vi "test_linear_interpolation.vi"() -> ()   [LabVIEW 2009]
doc: "Copyright (c) 2010 Stepan A. Baranov (stepan@baranov.su)\nAll rights reserved.\nweb-site: www.OCTLab.org"
uses:
  <vilib>/gmath/NI_Gmath.lvlib
  OCTLib_64.dll
panel:
  out "RSM_STAT final 2D array":dbl[](array[numeric])
  out "error out":errorcluster
  out "data Graph":dbl[][](graph)
  out "wavelengths Graph":dbl[][](graph)
  out "LabView final 2D array":dbl[](array[numeric])
  out "initial 2D array":dbl[](array[numeric])
  in  "stop":bool
  in  "index (row)":i32=1
  in  "Y":i32=9
  in  "X":i32=800
  in  "End wavelength":dbl=890.0
  in  "Start wavelength":dbl=800.0
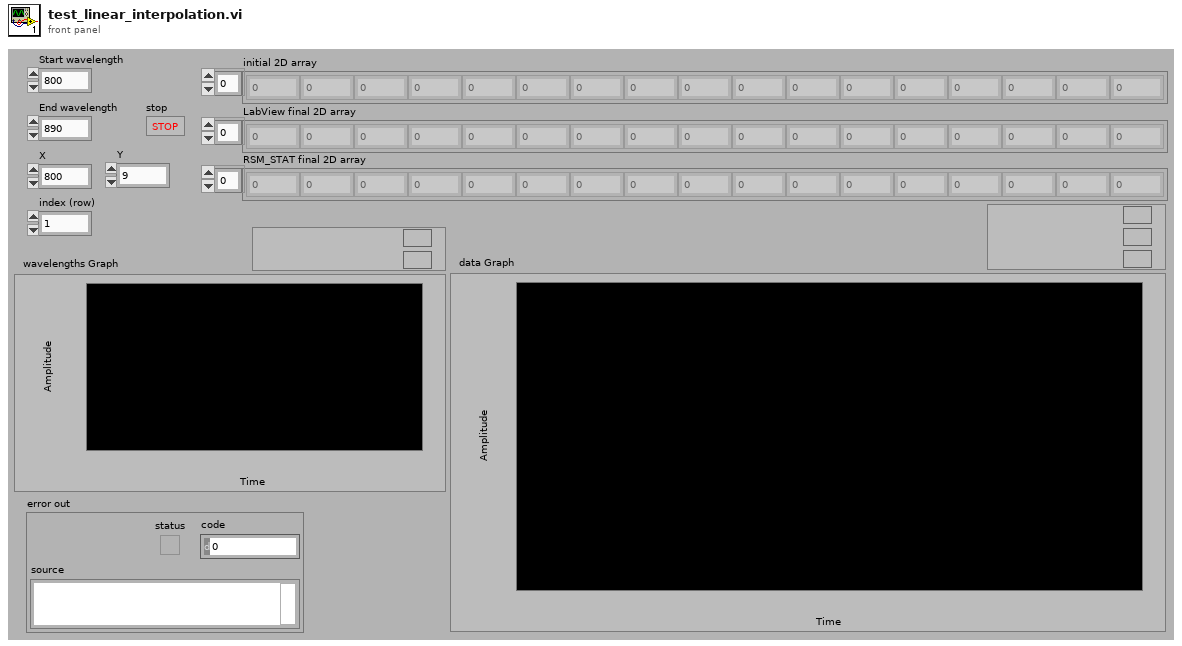
[diagram p1: front panel]
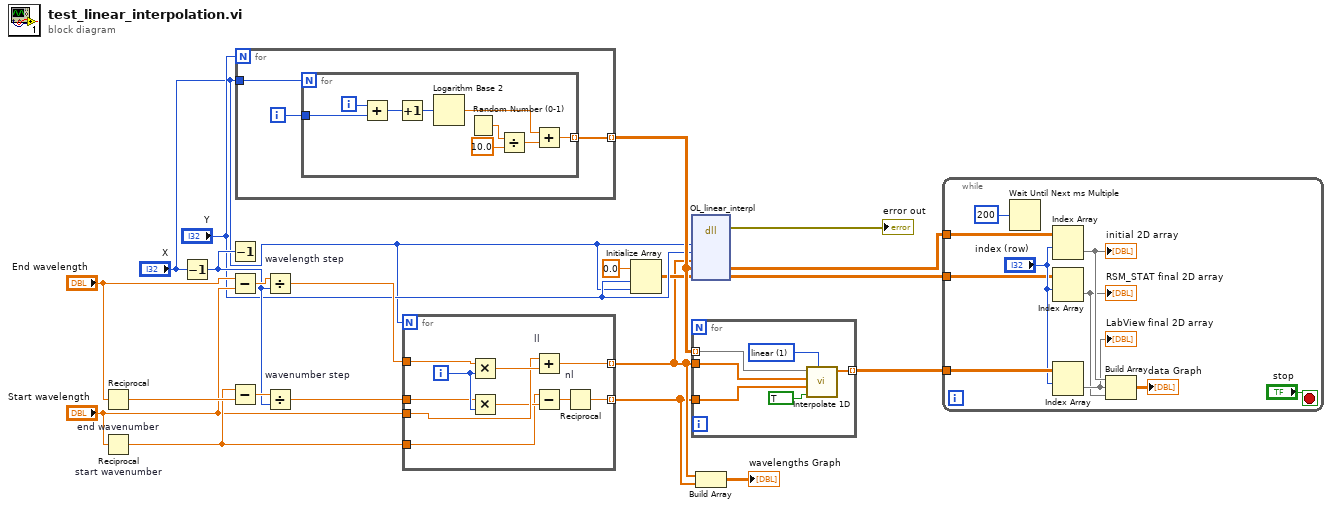
[diagram p0: block diagram]
diagram:
  n1 = Reciprocal "end wavenumber"(x="End wavelength") -> (1/x=w20:dbl)
  n2 = Reciprocal "start wavenumber"(x="Start wavelength") -> (1/x=w15:dbl)
  n3 = Decrement(x="X") -> (x-1=w18:i32)
  n4 = Decrement(x=w18) -> ()  [unwired: 1 out]
  n5 = Subtract(x="End wavelength", y="Start wavelength") -> (x-y=w21:dbl)
  n6 = Subtract(x=w15, y=w20) -> (x-y=w19:dbl)
  n7 = for {
    N: "Y" -> [_]
    tunnel: [w24] -> w11 mode=indexing
    tunnel: "X" -> [w23]
    i -> [w22]
    n8 = for {
      N: w23 -> [_]
      tunnel: [w25] -> w24 mode=indexing
      tunnel: w22 -> [w33]
      i -> [w32]
      n9 = Add(x=w32, y=w33) -> (x+y=w31:i32)
      n10 = Increment(x=w31) -> (x+1=w30:i32)
      n11 = Logarithm Base 2(1:w30) -> (0:w29:dbl)
      n12 = Random Number (0-1)() -> (number: 0 to 1=w28:dbl)
      n13 = Divide(x=w28, y=10.0) -> (x/y=w26:dbl)
      n14 = Add(x=w29, y=w26) -> (x+y=w25:dbl)
    }
  }
  n15 = Divide "wavelength step"(x=w21, y=w18) -> (x/y=w17:dbl)
  n16 = Divide "wavenumber step"(x=w19, y=w18) -> (x/y=w16:dbl)
  n17 = for {
    N: "X" -> [_]
    tunnel: w17 -> [w43]
    tunnel: "Start wavelength" -> [w41]
    tunnel: [w40] -> w3 mode=indexing
    tunnel: w16 -> [w38]
    tunnel: w15 -> [w35]
    tunnel: [w34] -> w2 mode=indexing
    i -> [w39]
    n18 = Multiply(x=w43, y=w39) -> (x*y=w42:dbl)
    n19 = Multiply(x=w38, y=w39) -> (x*y=w36:dbl)
    n20 = Add "ll"(x=w41, y=w42) -> (x+y=w40:dbl)
    n21 = Subtract(x=w35, y=w36) -> (x-y=w37:dbl)
    n22 = Reciprocal "nl"(x=w37) -> (1/x=w34:dbl)
  }
  n23 = Initialize Array(0.0 ("element"), "Y", "X") -> (w6:dbl[][])
  n24 = dll-call lib="OCTLib**.*" fn="OL_linear_interpl"("width"="X", "height"="Y", "spectrum"=w3, "in"=w11, "out"=w6) -> (error out=→"error out":errorcluster, "in"=w4:dbl[][], "out"=w10:dbl[][])  [unwired: 7 in, 1 out]
  n25 = for {
    tunnel: w11 -> [w49] mode=indexing
    tunnel: w3 -> [w48]
    tunnel: w2 -> [w47]
    tunnel: [w44] -> w1 mode=indexing
    w45 = 1 items=["nearest", "linear", "spline", "cubic Hermite", "Lagrange"] ("method")
    n26 = call <vilib>:"Interpolate 1D.vi"("method"=w45, "X is monotonic"=TRUE, "xi"=w47, "X"=w48, "Y"=w49) -> ("yi"=w44:dbl[])  [unwired: 4 in, 2 out]
  }
  n27 = Build Array(w3, w2) -> (→"wavelengths Graph":dbl[][])
  n28 = while {
    tunnel: w1 -> [w59]
    tunnel: w4 -> [w56]
    tunnel: w10 -> [w54]
    stop <- "stop" stop-if-true
    n29 = Wait Until Next ms Multiple(millisecond multiple=u32 200) -> ()  [unwired: 1 out]
    n30 = Index Array(array=w56, index (row)="index (row)") -> (element=w53:dbl[])  [unwired: 1 in]
    "initial 2D array" <- w53
    n31 = Index Array(array=w54, index (row)="index (row)") -> (element=w51:dbl[])  [unwired: 1 in]
    "RSM_STAT final 2D array" <- w51
    n32 = Index Array(array=w59, index (row)="index (row)") -> (element=w52:dbl[])  [unwired: 1 in]
    "LabView final 2D array" <- w52
    n33 = Build Array(w53, w52, w51) -> (→"data Graph":dbl[][])
  }
